vi "phaseVariables.vi"(0 "magVph":dbl, 1 "V ratio":dbl=100.0, 2 "phiVph":dbl, 3 "magIph":dbl, 4 "I ratio":dbl=40.0, 5 "phiIph":dbl) -> (7 "Magnitudes":T1)   [LabVIEW 2021]
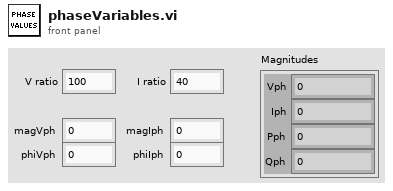
[diagram p1: front panel]
types:
  T1 = cluster{"Qph":dbl, "Pph":dbl, "Vph":dbl, "Iph":dbl}
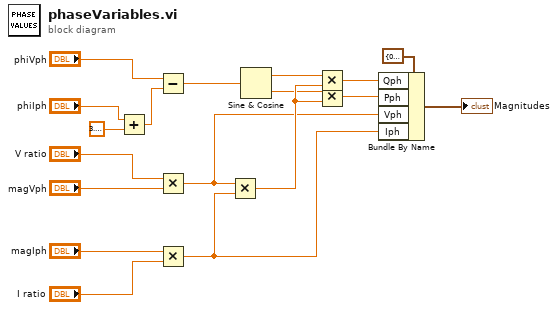
[diagram p0: block diagram]
diagram:
  n1 = Add(x="phiIph", y=3.141592653589793) -> (x+y=w2:dbl)
  n2 = Subtract(x="phiVph", y=w2) -> (x-y=w5:dbl)
  n3 = Multiply(x="V ratio", y="magVph") -> (x*y=w8:dbl)
  n4 = Multiply(x="magIph", y="I ratio") -> (x*y=w6:dbl)
  n5 = Multiply(x=w8, y=w6) -> (x*y=w18:dbl)
  n6 = Sine & Cosine(0:w5) -> (1:w17:dbl, 2:w16:dbl)
  n7 = Multiply(x=w17, y=w18) -> (x*y=w11:dbl)
  n8 = Multiply(x=w16, y=w18) -> (x*y=w10:dbl)
  n9 = Bundle By Name(cluster=T1 {"Qph"=0.0, "Pph"=0.0, "Vph"=0.0, "Iph"=0.0} ("Magnitudes"), "Qph"=w11, "Pph"=w10, "Vph"=w8, "Iph"=w6) -> (→"Magnitudes":T1)
